vi "Set Sif Comment.vi"(8 "error in (no error)":errorcluster, 11 "comment":string) -> (0 "error out":errorcluster, 2 "function return":u32, 3 "comment out":string)   [LabVIEW 2014, in "atmcd32d.lvlib"]
doc: "unsigned int WINAPI SetSifComment(char * comment);"
uses:
  atmcd32d.lvlib
  atmcd32d.dll
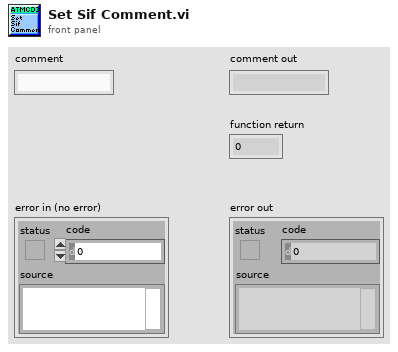
[diagram p1: front panel]
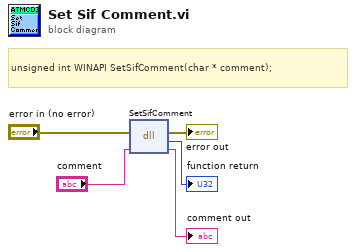
[diagram p0: block diagram]
diagram:
  # "unsigned int WINAPI SetSifComment(char * comment);"
  n1 = dll-call lib="C:/Users/Bakir/Documents/Lambda2-Testing/lib/Andorlib/atmcd32d.*" fn="SetSifComment"(error in="error in (no error)", "comment"="comment") -> (error out=→"error out":errorcluster, →"function return":u32, "comment"=→"comment out":string)  [unwired: 2 in, 1 out]
